vi "Limit Check.vi"(2 "Limit the \nOutput":bool, 3 "Limit":dbl[][](array[numeric]), 4 "Fault Id In":T1, 5 "Input":dbl[](array[numeric])) -> (0 "Within Limit":bool[](array[boolean]), 1 "Output":dbl[](array[numeric]))   [LabVIEW 2013]
uses:
  Fault Id.ctl
  Fault Type.ctl
  Data Access Objects/Metadata/LBCB Number.ctl
  Space Type.ctl
  Faults List Actions.ctl
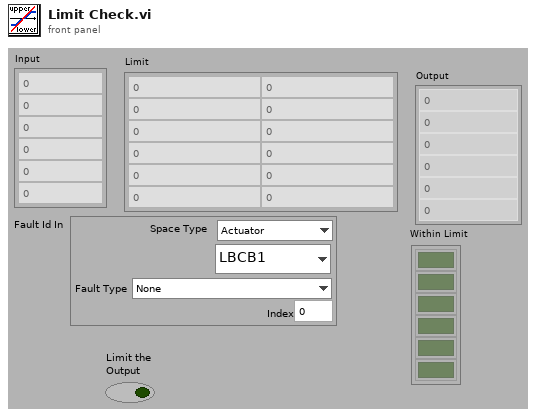
[diagram p1: front panel]
types:
  T1 = typedef "Fault Id.ctl" = cluster{"Fault Type":T2, "LBCB Number":T3, "Index":u32, "Space Type":T4}
  T2 = typedef "Fault Type.ctl" = enum16{"None", "Command", "Displacement", "Force", "Increment"}
  T3 = typedef "LBCB Number.ctl" = enum16{"LBCB1", "LBCB2"}
  T4 = typedef "Space Type.ctl" = enum16{"Actuator", "Cartesian"}
  T5 = typedef "Faults List Actions.ctl" = enum16{"Init", "Add", "Remove", "Get List"}
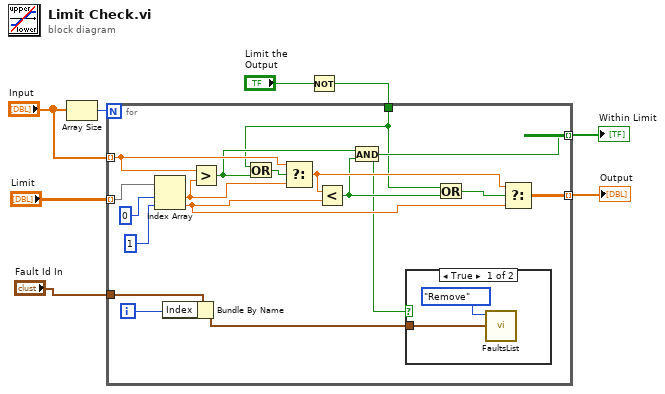
[diagram p0: block diagram]
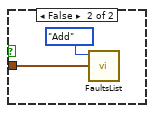
[diagram p2: hidden frame]
diagram:
  n1 = Array Size(array="Input") -> (size(s)=w8:i32)
  n2 = Not(x="Limit the \nOutput") -> (.not. x?=w1:bool)
  n3 = for {
    N: w8 -> [_]
    tunnel: "Input" -> [w21] mode=indexing
    tunnel: [w25] -> w6 mode=indexing
    tunnel: "Limit" -> [w22] mode=indexing
    tunnel: "Fault Id In" -> [w15]
    tunnel: [w12] -> w4 mode=indexing
    tunnel: w1 -> [w9]
    i -> [w13]
    n4 = Index Array(array=w22, index #1=0, index #2=1) -> (element #1=w20:dbl, element #2=w19:dbl)
    n5 = Bundle By Name(cluster=w15, "Index"=w13) -> (w14:T1)
    n6 = Greater?(x=w21, y=w20) -> (0:w17:bool)
    n7 = Or(x=w9, y=w17) -> (x .or. y?=w10:bool)
    n8 = Select(t=w21, s=w10, f=w20) -> (s? t:f=w18:dbl)
    n9 = Less?(x=w18, y=w19) -> (x < y?=w16:bool)
    n10 = And(x=w17, y=w16) -> (x .and. y?=w12:bool)
    n11 = case shown="True" w12 {
      tunnel: w14 -> [w26 w28]
      frame True {
        n12 = call "FaultsList.vi"("Fault Id In"=w26, "Limits List Actions"=Faults_List_Actions."Remove") -> ()  [unwired: 1 in, 9 out]
      }
      frame False {
        n13 = call "FaultsList.vi"("Fault Id In"=w28, "Limits List Actions"=Faults_List_Actions."Add") -> ()  [unwired: 1 in, 9 out]
      }
    }
    n14 = Or(x=w9, y=w16) -> (x .or. y?=w11:bool)
    n15 = Select(t=w18, s=w11, f=w19) -> (s? t:f=w25:dbl)
  }
  "Output" <- w6
  "Within Limit" <- w4
